vi "NtoSVXXXX.vi"(1 "Numeric":dbl) -> (0 "String":string)   [LabVIEW 2011]
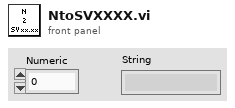
[diagram p1: front panel]
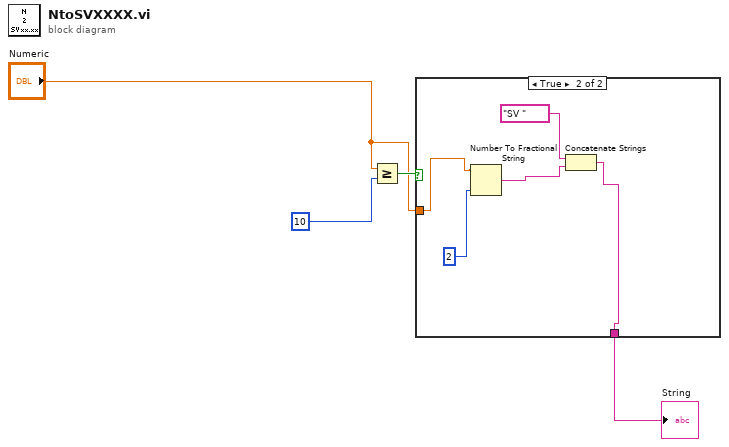
[diagram p0: block diagram]
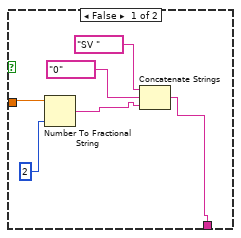
[diagram p2: hidden frame]
diagram:
  n1 = Greater Or Equal?(x="Numeric", y=10) -> (x >= y?=w3:bool)
  n2 = case shown="True" w3 {
    tunnel: [w6 w12] -> w1
    tunnel: "Numeric" -> [w5 w11]
    frame False {
      n3 = Number To Fractional String(number=w5, precision (6)=2) -> (F-format string=w9:string)  [unwired: 2 in]
      n4 = Concatenate Strings("SV ", "0", w9) -> (w6:string)
    }
    frame True {
      n5 = Number To Fractional String(number=w11, precision (6)=2) -> (F-format string=w14:string)  [unwired: 2 in]
      n6 = Concatenate Strings("SV ", w14) -> (w12:string)
    }
  }
  "String" <- w1
